vi "Climb Teleop.vi"(11 "Cluster":T1) -> ()   [LabVIEW 2018]
uses:
  Support Code/Joystick Vals.ctl
  Implementation/Climb Operations.ctl
  Drive/Implementation/Drive Operations.ctl
  Support Code/Rhino States.ctl
  Framework/Robot Global Data.vi
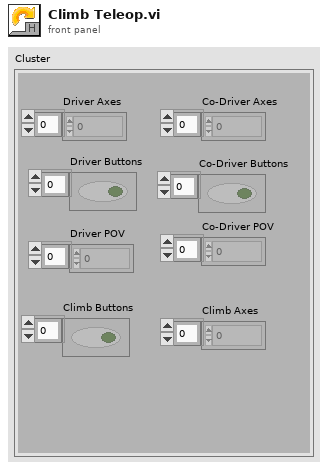
[diagram p1: front panel]
types:
  T1 = typedef "Joystick Vals.ctl" = cluster{"Driver Axes":dbl[], "Co-Driver Axes":dbl[], "Driver Buttons":bool[], "Co-Driver Buttons":bool[], "Driver POV":i16[], "Co-Driver POV":i16[], "Climb Buttons":bool[], "Climb Axes":dbl[]}
  T2 = typedef "Rhino States.ctl" = enum16{"Step 1: Climb", "Step 2: Drive Forwards", "Step 3: Pull Stilts Up", "Step 4: Drive and Tilt"}
  T3 = typedef "Climb Operations.ctl" = enum16{"Reserve", "Read Current", "Immediate", "Ready", "Auto-Climb", "Reset/Turbo-Tilt", "Manual Climb"}
  T4 = typedef "Drive Operations.ctl" = enum16{"Reserve", "Read Current", "Immediate", "J-Turn", "Play Back From Log", "Auto-Align"}
  T5 = cluster{"Reverse (T) / Normal (F)":bool, "Power Scaling (1=Normal) ":dbl, "Deadband Value":dbl}
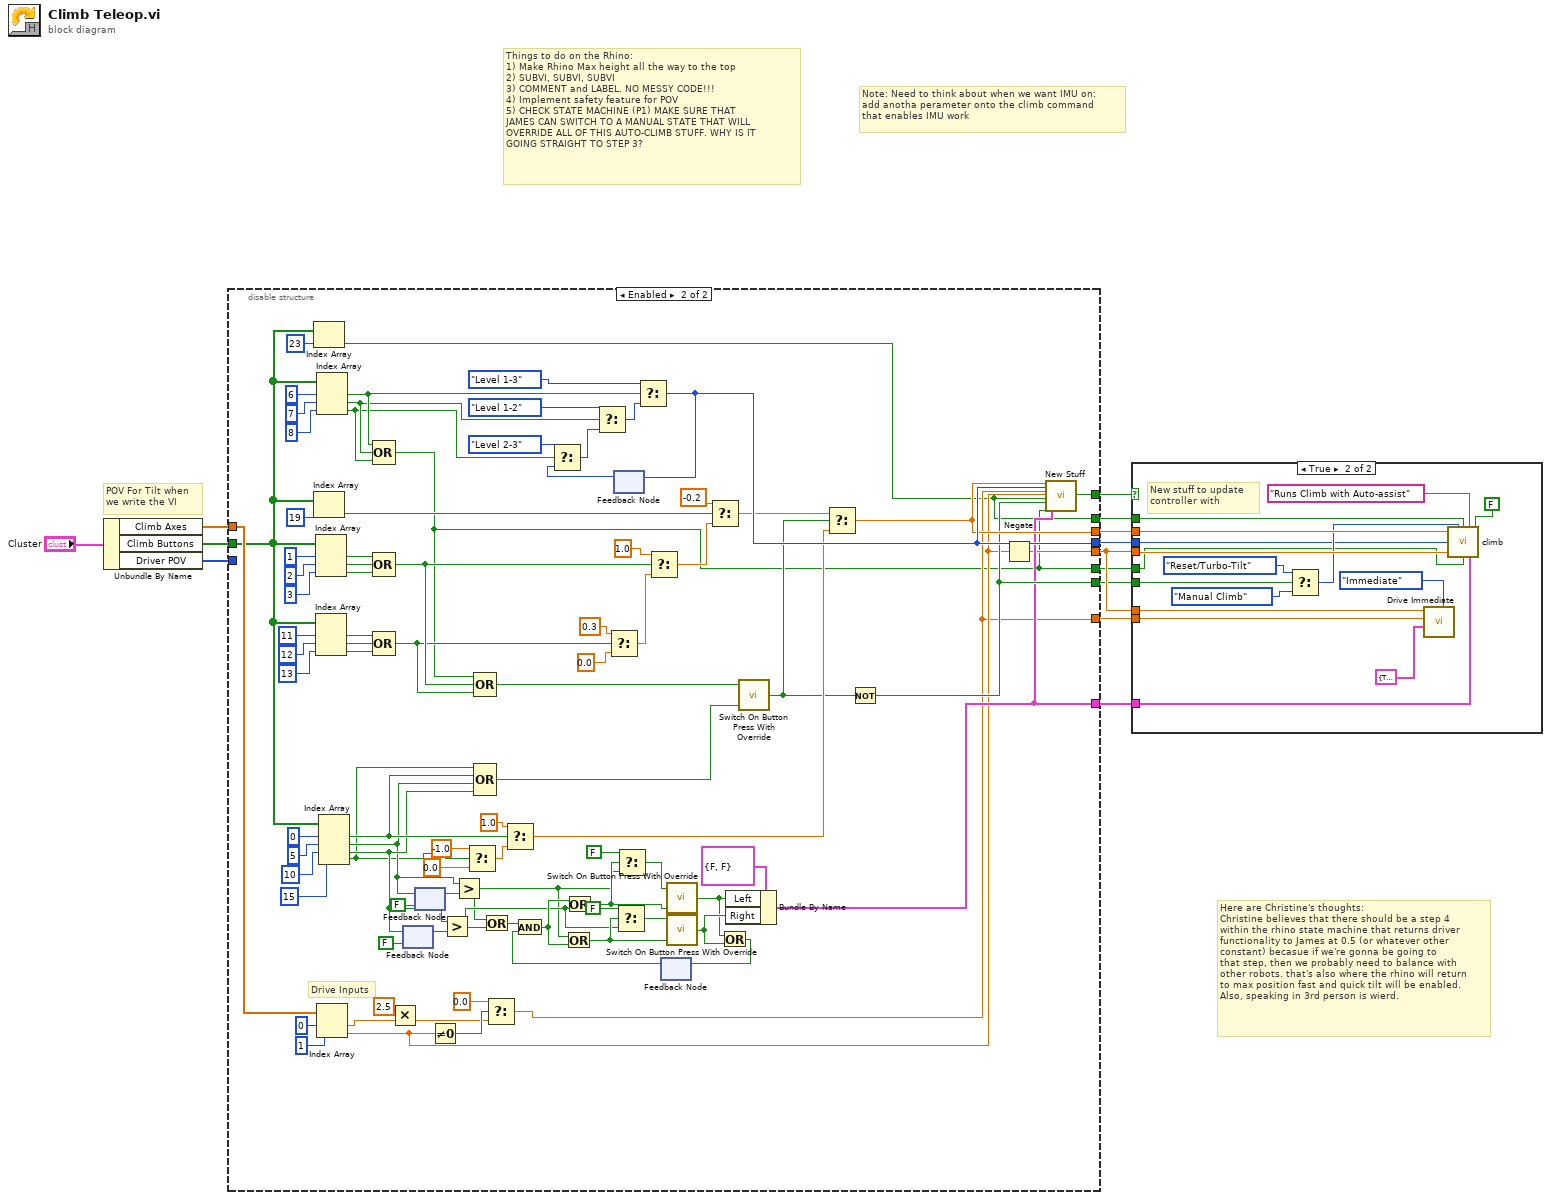
[diagram p0: block diagram]
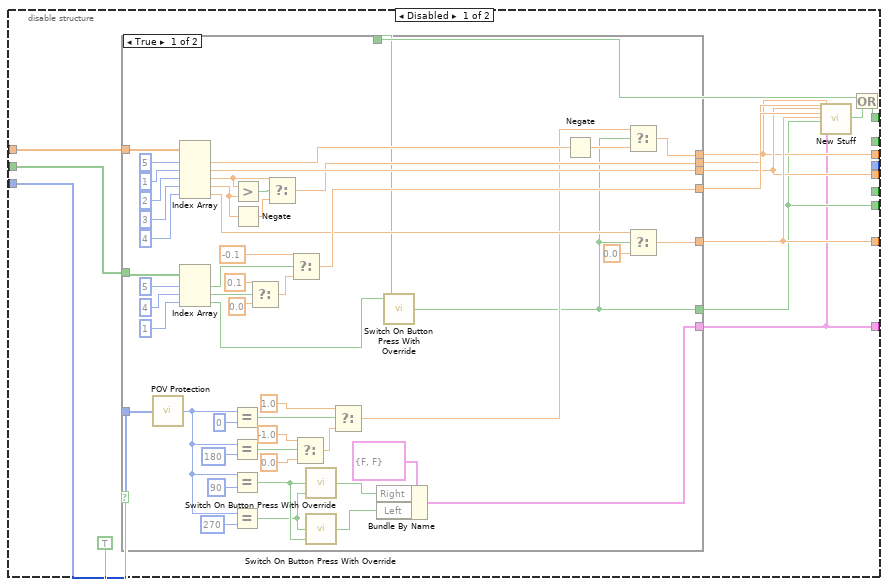
[diagram p2: hidden frame]
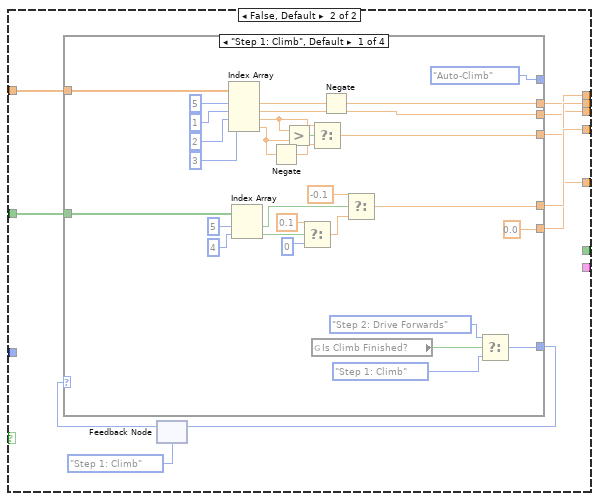
[diagram p3: hidden frame]
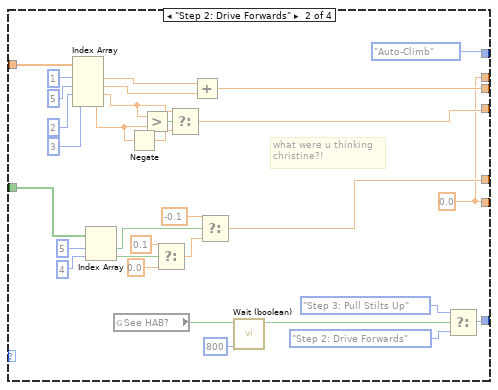
[diagram p4: hidden frame]
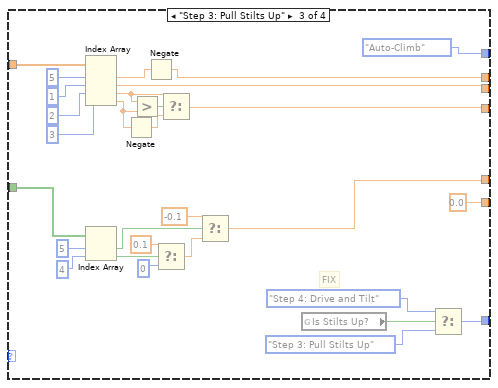
[diagram p5: hidden frame]
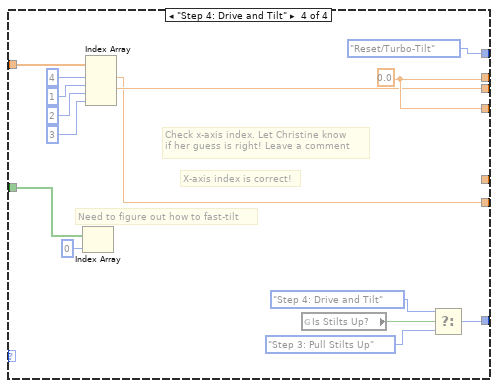
[diagram p6: hidden frame]
diagram:
  # "Note: Need to think about when we want IMU on:\nadd anotha perameter onto the climb command\nthat enables IMU work"
  # "Things to do on the Rhino:\n1) Make Rhino Max height all the way to the top\n2) SUBVI, SUBVI, SUBVI\n3) COMMENT and LABEL. NO MESSY CODE!!!\n4) Implement safety feature for POV\n5) CHECK STATE MACHINE (P1) MAKE SURE THAT\nJAMES CAN SWITCH TO A MANUAL STATE THAT WILL\nOVERRIDE ALL OF THIS AUTO-CLIMB STUFF. WHY IS IT\nGOING STRAIGHT TO STEP 3?"
  # "Here are Christine's thoughts:\nChristine believes that there should be a step 4\nwithin the rhino state machine that returns driver\nfunctionality to James at 0.5 (or whatever other \nconstant) becasue if we're gonna be going to \nthat step, then we probably need to balance with\nother robots. that's also where the rhino will return \nto max position fast and quick tilt will be enabled.\nAlso, speaking in 3rd person is wierd."
  # "POV For Tilt when\nwe write the VI"
  n1 = Unbundle By Name("Cluster") -> ("Climb Axes"=w11:dbl[], "Climb Buttons"=w12:bool[], "Driver POV"=w10:i16[])
  n2 = disable-structure shown="Enabled" {
    disable-tunnel: w12 -> [w28 w245]
    disable-tunnel: w11 -> [w27 w267]
    disable-tunnel: w10 -> [w25 _]
    disable-tunnel: [w24 w224] -> w9
    disable-tunnel: [w22 w228] -> w8
    disable-tunnel: [w20 w243] -> w7
    disable-tunnel: [w19 w230] -> w6
    disable-tunnel: [w18 w229] -> w5
    disable-tunnel: [w15 w255] -> w4
    disable-tunnel: [_ w254] -> w3
    disable-tunnel: [_ w196] -> w2
    disable-tunnel: [_ w203] -> w1
    frame Disabled {
      n3 = case shown="True" TRUE {
        tunnel: w28 -> [w58 w89]
        tunnel: [w60 w88] -> w23
        tunnel: w27 -> [w59 w85]
        tunnel: [w61 w84] -> w21
        tunnel: [w51 w83] -> w20
        tunnel: [w62 w82] -> w22
        tunnel: [w56 w80] -> w24
        tunnel: w25 -> [w50 _]
        tunnel: [w30 _] -> w19
        tunnel: [w34 _] -> w18
        tunnel: w14 -> [w29 _]
        frame True {
          n4 = call "POV Protection.vi"("Array"=w50) -> ("s? t:f"=w38:i32)
          n5 = Index Array(array=w59, index #1=5 ("index"), index #2=1 ("index"), index #3=2 ("index"), index #4=3 ("index"), index #5=4 ("index")) -> (element #1=w64:dbl, element #2=w62:dbl, element #3=w71:dbl, element #4=w72:dbl, element #5=w53:dbl)
          n6 = Index Array(array=w58, index #1=5 ("index"), index #2=4 ("index"), index #3=1 ("index")) -> (element #1=w79:bool, element #2=w77:bool, element #3=w31:bool)
          n7 = Equal?(x=w38, y=0) -> (x = y?=w47:bool)
          n8 = Equal?(x=w38, y=180) -> (x = y?=w46:bool)
          n9 = Equal?(x=w38, y=90) -> (x = y?=w33:bool)
          n10 = Equal?(x=w38, y=270) -> (x = y?=w32:bool)
          n11 = Greater?(x=w71, y=w72) -> (0:w70:bool)
          n12 = Negate(x=w72) -> (-x=w69:dbl)
          n13 = Select(t=0.1, s=w77, f=0.0) -> (s? t:f=w78:dbl)
          n14 = Select(t=w71, s=w70, f=w69) -> (s? t:f=w61:dbl)
          n15 = Select(t=-0.1, s=w79, f=w78) -> (s? t:f=w60:dbl)
          n16 = Select(t=-1.0, s=w46, f=0.0) -> (s? t:f=w43:dbl)
          n17 = call "Switch On Button Press With Override.vi"("Override False"=w32, "Button"=w33) -> ("Output"=w37:bool)  [unwired: 1 in]
          n18 = call "Switch On Button Press With Override.vi"("Override False"=w33, "Button"=w32) -> ("Output"=w36:bool)  [unwired: 1 in]
          n19 = Select(t=1.0, s=w47, f=w43) -> (s? t:f=w41:dbl)
          n20 = Bundle By Name(cluster=cluster{"Right":bool, "Left":bool} {"Right"=FALSE, "Left"=FALSE} ("input cluster"), "Right"=w37, "Left"=w36) -> (w34:cluster{"Right":bool, "Left":bool})
          n21 = call "Switch On Button Press With Override.vi"("Override False"=w29, "Override True"=w31) -> ("Output"=w30:bool)  [unwired: 1 in]
          n22 = Negate(x=w64) -> (-x=w52:dbl)
          n23 = Select(t=w41, s=w30, f=w52) -> (s? t:f=w51:dbl)
          n24 = Select(t=w53, s=w30, f=0.0) -> (s? t:f=w56:dbl)
        }
        frame False, Default {
          n25 = feedback #1(Rhino_States."Step 1: Climb") -> (w87:T2)
          n26 = case shown="\"Step 1: Climb\", Default" w87 {
            tunnel: w89 -> [w113 w140 w172 w181]
            tunnel: [w110 w139 w169 _] -> w88
            tunnel: [w108 w135 w156 w188] -> w86
            tunnel: w85 -> [w103 w149 w164 w189]
            tunnel: [w98 w125 w157 w184] -> w84
            tunnel: [w91 w120 w151 w184] -> w83
            tunnel: [w96 w121 w163 w183] -> w82
            tunnel: [0.0 w120 0.0 w182] -> w80
            tunnel: [Climb_Operations."Auto-Climb" ("Operation") Climb_Operations."Auto-Climb" ("Operation") Climb_Operations."Auto-Climb" ("Operation") Climb_Operations."Reset/Turbo-Tilt" ("Operation")] -> _
            frame "Step 1: Climb", Default {
              n27 = Index Array(array=w103, index #1=5 ("index"), index #2=1 ("index"), index #3=2 ("index"), index #4=3 ("index")) -> (element #1=w97:dbl, element #2=w96:dbl, element #3=w106:dbl, element #4=w107:dbl)
              n28 = Index Array(array=w113, index #1=5 ("index"), index #2=4 ("index")) -> (element #1=w118:bool, element #2=w116:bool)
              n29 = Negate(x=w107) -> (-x=w104:dbl)
              n30 = Greater?(x=w106, y=w107) -> (0:w105:bool)
              n31 = Select(t=0.1, s=w116, f=0) -> (s? t:f=w117:dbl)
              n32 = Select(t=w106, s=w105, f=w104) -> (s? t:f=w98:dbl)
              n33 = global read "Robot Global Data.vi" "Is Climb Finished?"() -> (w109:bool)
              n34 = Negate(x=w97) -> (-x=w91:dbl)
              n35 = Select(t=-0.1, s=w118, f=w117) -> (s? t:f=w110:dbl)
              n36 = Select(t=Rhino_States."Step 2: Drive Forwards", s=w109, f=Rhino_States."Step 1: Climb") -> (s? t:f=w108:T2)
            }
            frame "Step 2: Drive Forwards" {
              w120 = 0.0
              # "what were u thinking\nchristine?!"
              n37 = Index Array(array=w149, index #1=1, index #2=5, index #3=2 ("index"), index #4=3 ("index")) -> (element #1=w138:dbl, element #2=w137:dbl, element #3=w127:dbl, element #4=w126:dbl)
              n38 = Index Array(array=w140, index #1=5 ("index"), index #2=4 ("index")) -> (element #1=w146:bool, element #2=w144:bool)
              n39 = global read "Robot Global Data.vi" "See HAB?"() -> (w123:bool)
              n40 = Negate(x=w126) -> (-x=w130:dbl)
              n41 = Greater?(x=w127, y=w126) -> (0:w131:bool)
              n42 = Select(t=0.1, s=w144, f=0.0) -> (s? t:f=w145:dbl)
              n43 = Select(t=w127, s=w131, f=w130) -> (s? t:f=w125:dbl)
              n44 = Add(x=w138, y=w137) -> (x+y=w121:dbl)
              n45 = Select(t=-0.1, s=w146, f=w145) -> (s? t:f=w139:dbl)
              n46 = call "Wait (boolean).vi"("Time to wait (ms)"=800, "In"=w123) -> ("Out"=w122:bool)  [unwired: 9 in]
              n47 = Select(t=Rhino_States."Step 3: Pull Stilts Up", s=w122, f=Rhino_States."Step 2: Drive Forwards") -> (s? t:f=w135:T2)
            }
            frame "Step 3: Pull Stilts Up" {
              # "FIX"
              n48 = Index Array(array=w164, index #1=5 ("index"), index #2=1 ("index"), index #3=2 ("index"), index #4=3 ("index")) -> (element #1=w162:dbl, element #2=w163:dbl, element #3=w158:dbl, element #4=w159:dbl)
              n49 = Index Array(array=w172, index #1=5 ("index"), index #2=4 ("index")) -> (element #1=w178:bool, element #2=w176:bool)
              n50 = Negate(x=w159) -> (-x=w160:dbl)
              n51 = Greater?(x=w158, y=w159) -> (0:w161:bool)
              n52 = Negate(x=w162) -> (-x=w151:dbl)
              n53 = Select(t=0.1, s=w176, f=0) -> (s? t:f=w177:dbl)
              n54 = Select(t=w158, s=w161, f=w160) -> (s? t:f=w157:dbl)
              n55 = Select(t=-0.1, s=w178, f=w177) -> (s? t:f=w169:dbl)
              n56 = global read "Robot Global Data.vi" "Is Stilts Up?"() -> (w155:bool)
              n57 = Select(t=Rhino_States."Step 4: Drive and Tilt", s=w155, f=Rhino_States."Step 3: Pull Stilts Up") -> (s? t:f=w156:T2)
            }
            frame "Step 4: Drive and Tilt" {
              w184 = 0.0
              # "X-axis index is correct!"
              # "Need to figure out how to fast-tilt"
              # "Check x-axis index. Let Christine know \nif her guess is right! Leave a comment"
              n58 = Index Array(array=w181, index=0) -> ()  [unwired: 1 out]
              n59 = Index Array(array=w189, index #1=4 ("index"), index #2=1 ("index"), index #3=2 ("index"), index #4=3 ("index")) -> (element #1=w182:dbl, element #2=w183:dbl)  [unwired: 2 out]
              n60 = global read "Robot Global Data.vi" "Is Stilts Up?"() -> (w187:bool)
              n61 = Select(t=Rhino_States."Step 4: Drive and Tilt", s=w187, f=Rhino_States."Step 3: Pull Stilts Up") -> (s? t:f=w188:T2)
            }
          }
          n62 = feedback-in #1(w86) -> ()
        }
      }
      n63 = call "New Stuff.vi"("Variant"=w21, "Variant 2"=w22, "Variant 4"=w23, "Variant 3"=w24, "Variant 16"=w19, "Variant 5"=w20, "Variant 14"=w18) -> ("Variant 15"=w17:variant, "x != y?"=w16:bool)  [unwired: 19 in]
      n64 = Or(y=w16) -> (x=w14:bool, x .or. y?=w15:bool)
    }
    frame Enabled {
      # "Drive Inputs"
      n65 = Index Array(array=w245, index=23) -> (element=w196:bool)
      n66 = Index Array(array=w245, index=19) -> (element=w250:bool)
      n67 = Index Array(array=w245, index #1=1 ("index"), index #2=2 ("index"), index #3=3 ("index")) -> (element #1=w279:bool, element #2=w278:bool, element #3=w277:bool)
      n68 = Index Array(array=w245, index #1=11 ("index"), index #2=12 ("index"), index #3=13 ("index")) -> (element #1=w273:bool, element #2=w272:bool, element #3=w271:bool)
      n69 = Index Array(array=w245, index #1=6 ("index"), index #2=7 ("index"), index #3=8 ("index")) -> (element #1=w242:bool, element #2=w241:bool, element #3=w240:bool)
      n70 = Index Array(array=w267, index #1=0 ("index"), index #2=1 ("index")) -> (element #1=w223:dbl, element #2=w225:dbl)
      n71 = Index Array(array=w245, index #1=0 ("index"), index #2=5 ("index"), index #3=10 ("index"), index #4=15 ("index")) -> (element #1=w237:bool, element #2=w204:bool, element #3=w208:bool, element #4=w198:bool)
      n72 = Compound Arithmetic op=OR(w242, w241, w240) -> (w203:bool)
      n73 = Compound Arithmetic op=OR(w279, w278, w277) -> (w239:bool)
      n74 = Compound Arithmetic op=OR(w273, w272, w271) -> (w238:bool)
      n75 = Multiply(x=2.5, y=w223) -> (x*y=w195:dbl)
      n76 = feedback-in #2(w208) -> ()
      n77 = feedback #2(FALSE ("Boolean")) -> (w209:bool)
      n78 = feedback #3(FALSE ("Boolean")) -> (w206:bool)
      n79 = feedback-in #3(w204) -> ()
      n80 = Not Equal To 0?(x=w225) -> (x != 0?=w227:bool)
      n81 = Greater?(x=w208, y=w209) -> (0:w207:bool)
      n82 = Greater?(x=w204, y=w206) -> (0:w201:bool)
      n83 = Select(t=-1.0, s=w198, f=0.0) -> (s? t:f=w199:dbl)
      n84 = Compound Arithmetic op=OR(w203, w239, w238) -> (w232:bool)
      n85 = Compound Arithmetic op=OR(w198, w237, w204, w208) -> (w231:bool)
      n86 = Or(x=w201, y=w207) -> (x .or. y?=w219:bool)
      n87 = Select(t=0.0, s=w227, f=w195) -> (s? t:f=w224:dbl)
      n88 = Select(t=1.0, s=w237, f=w199) -> (s? t:f=w234:dbl)
      n89 = Select(t=0.3, s=w238, f=0.0) -> (s? t:f=w270:dbl)
      n90 = feedback #4() -> (w256:enum16{"Level 1-3", "Level 1-2", "Level 2-3"})  [unwired: 1 in]
      n91 = Select(t=enum16{"Level 1-3", "Level 1-2", "Level 2-3"}."Level 2-3" ("Enum"), s=w240, f=w256) -> (s? t:f=w258:enum16{"Level 1-3", "Level 1-2", "Level 2-3"})
      n92 = Select(t=enum16{"Level 1-3", "Level 1-2", "Level 2-3"}."Level 1-2" ("Enum"), s=w241, f=w258) -> (s? t:f=w260:enum16{"Level 1-3", "Level 1-2", "Level 2-3"})
      n93 = Select(t=enum16{"Level 1-3", "Level 1-2", "Level 2-3"}."Level 1-3" ("Enum"), s=w242, f=w260) -> (s? t:f=w254:enum16{"Level 1-3", "Level 1-2", "Level 2-3"})
      n94 = feedback-in #4(w254) -> ()
      n95 = Select(t=1.0, s=w239, f=w270) -> (s? t:f=w251:dbl)
      n96 = feedback #5() -> (w218:bool)  [unwired: 1 in]
      n97 = And(x=w219, y=w218) -> (x .and. y?=w217:bool)
      n98 = Or(x=w201, y=w217) -> (x .or. y?=w212:bool)
      n99 = Or(x=w217, y=w207) -> (x .or. y?=w216:bool)
      n100 = Select(t=FALSE, s=w212, f=w207) -> (s? t:f=w211:bool)
      n101 = Select(t=FALSE, s=w216, f=w201) -> (s? t:f=w214:bool)
      n102 = call "Switch On Button Press With Override.vi"("Override False"=w216, "Override True"=w214) -> ("Output"=w221:bool)  [unwired: 1 in]
      n103 = call "Switch On Button Press With Override.vi"("Override False"=w212, "Override True"=w211) -> ("Output"=w222:bool)  [unwired: 1 in]
      n104 = Select(t=-0.2, s=w250, f=w251) -> (s? t:f=w235:dbl)
      n105 = Or(x=w221, y=w222) -> (x .or. y?=w220:bool)
      n106 = feedback-in #5(w220) -> ()
      n107 = Bundle By Name(cluster=cluster{"Right":bool, "Left":bool} {"Right"=FALSE, "Left"=FALSE} ("input cluster"), "Left"=w221, "Right"=w222) -> (w229:cluster{"Right":bool, "Left":bool})
      n108 = call "Switch On Button Press With Override.vi"("Override False"=w231, "Override True"=w232) -> ("Output"=w233:bool)  [unwired: 1 in]
      n109 = Select(t=w235, s=w233, f=w234) -> (s? t:f=w243:dbl)
      n110 = Not(x=w233) -> (.not. x?=w230:bool)
      n111 = Negate(x=w225) -> (-x=w228:dbl)
      n112 = call "New Stuff.vi"("Variant"=w243, "Variant 2"=w254, "Variant 4"=w224, "Variant 3"=w225, "Variant 16"=w196, "Variant 15"=w230, "Variant 7"=w203, "Variant 14"=w229) -> ("x != y?"=w255:bool)  [unwired: 19 in]
    }
  }
  n113 = case shown="True" w4 {
    tunnel: w7 -> [_ w295]
    tunnel: w8 -> [_ w299]
    tunnel: w8 -> [_ w297]
    tunnel: w9 -> [_ w296]
    tunnel: w6 -> [_ w292]
    tunnel: w5 -> [_ w289]
    tunnel: w3 -> [_ w288]
    tunnel: w2 -> [_ w287]
    tunnel: w1 -> [_ w285]
    frame False {
      # "Nothing new to send"
    }
    frame True {
      # "New stuff to update \ncontroller with"
      n114 = Select(t=Climb_Operations."Reset/Turbo-Tilt" ("Operation"), s=w292, f=Climb_Operations."Manual Climb" ("Operation")) -> (s? t:f=w291:T3)
      n115 = call "Drive Immediate.vi"("Operation"=Drive_Operations."Immediate", "Modifiers"=T5 {"Reverse (T) / Normal (F)"=TRUE, "Power Scaling (1=Normal) "=0.275, "Deadband Value"=0.05}, "Right Setpoint (Turning)"=w296, "Left Setpoint (Power)"=w297) -> ()  [unwired: 7 in, 1 out]
      n116 = call "climb.vi"("Setpoint ARM"=w295, "Operation"=w291, "Reset"=w287, "Description"="Runs Climb with Auto-assist", "Defense mode?"=FALSE, "Enum"=w288, "Setpoint WHEELS"=w299, "New Pos?"=w285, "Speedy Tilt"=w289) -> ()  [unwired: 6 in, 1 out]
    }
  }
